vi "Varint Decoder boolean.vi"(7 "Optional":bool, 8 "error in (no error)":errorcluster, 9 "Array":u8[](array[numeric]) format="%02x", 10 "Key":i32=-1) -> (0 "error out":errorcluster, 1 "array w/ subset deleted":u8[](array[numeric]), 2 "Read Key":i32, 3 "bool":bool)   [LabVIEW 2021]
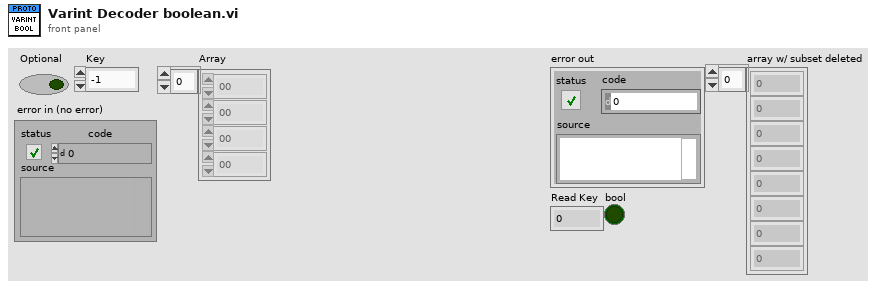
[diagram p1: front panel]
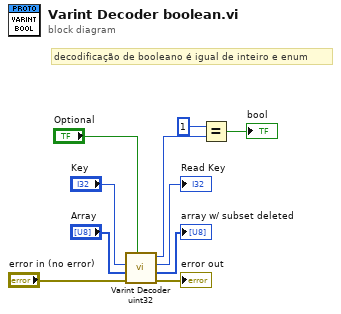
[diagram p0: block diagram]
diagram:
  # "decodificação de booleano é igual de inteiro e enum"
  n1 = call "Varint Decoder uint32.vi"("Optional"="Optional", "error in (no error)"="error in (no error)", "Array"="Array", "Key"="Key") -> ("error out"=→"error out":errorcluster, "array w/ subset deleted"=→"array w/ subset deleted":u8[], "Read Key"=→"Read Key":i32, "Varint"=w3:u32)  [unwired: 4 in]
  n2 = Equal?(x=u32 1, y=w3) -> (x = y?=→"bool":bool)
